vi "Mandatory Field Missing.vi"(8 "error in":errorcluster, 10 "Field Name":string, 11 "Object Type Base":refnum<class "Object Type Base.lvclass">) -> (0 "error out":errorcluster)   [LabVIEW 2024, in "EDS.lvlib" / "Object Type Base.lvclass"]
uses:
  Object Type Base.lvclass
  Object Type Base.lvclass/Object Type Base.ctl
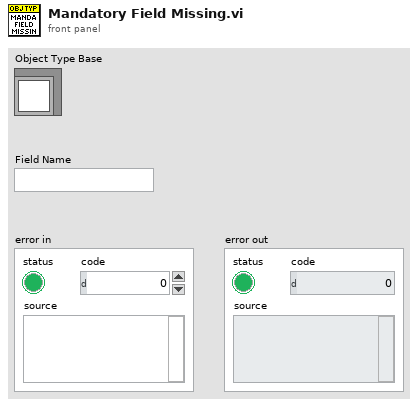
[diagram p1: front panel]
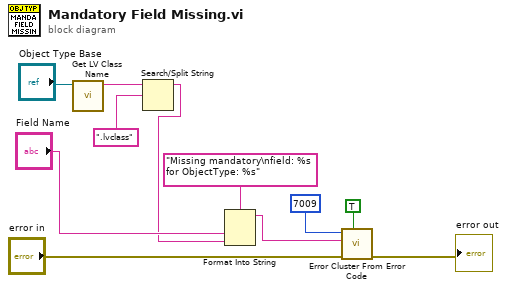
[diagram p0: block diagram]
diagram:
  n1 = call <vilib>:"Get LV Class Name.vi"("object"="Object Type Base") -> ("class name"=w3:string)  [unwired: 9 in, 1 out]
  n2 = Search/Split String(string=w3, search string/char (-)=".lvclass") -> (substring before match=w1:string)  [unwired: 1 in, 2 out]
  n3 = Format Into String(format string="Missing mandatory\nfield: %s for ObjectType: %s", "Field Name", w1) -> (resulting string=w7:string)  [unwired: 2 in, 1 out]
  n4 = call <vilib>:"Error Cluster From Error Code.vi"("show call chain? (False)"=TRUE, "error in (no error)"="error in", "error message (\"\")"=w7, "error code (0)"=7009) -> ("error out"=→"error out":errorcluster)  [unwired: 5 in]
